vi "Repack Color to Color Array.vi"(11 "Pixel Data":T1={"A"=[0, 0, 0, 0, 0, 0, 0, 0], "R/H"=[0, 0, 0, 0, 0, 0, 0, 0], "G/S"=[0, 0, 0, 0, 0, 0, 0, 0], "B/L"=[0, 0, 0, 0, 0, 0, 0, 0]}) -> (3 "Output array U32x8":u32[](array[numeric]))   [LabVIEW 2017, in "NI_VDM_FPGA_Basics.lvlib"]
uses:
  <vilib>/visionFPGA/NI_VDM_FPGA_Basics.lvlib
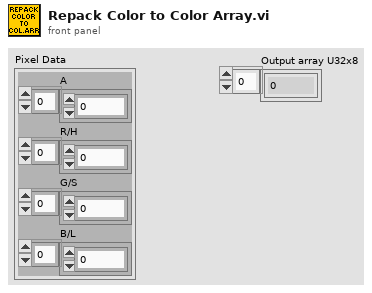
[diagram p1: front panel]
types:
  T1 = cluster{"A":u8[], "R/H":u8[], "G/S":u8[], "B/L":u8[]}
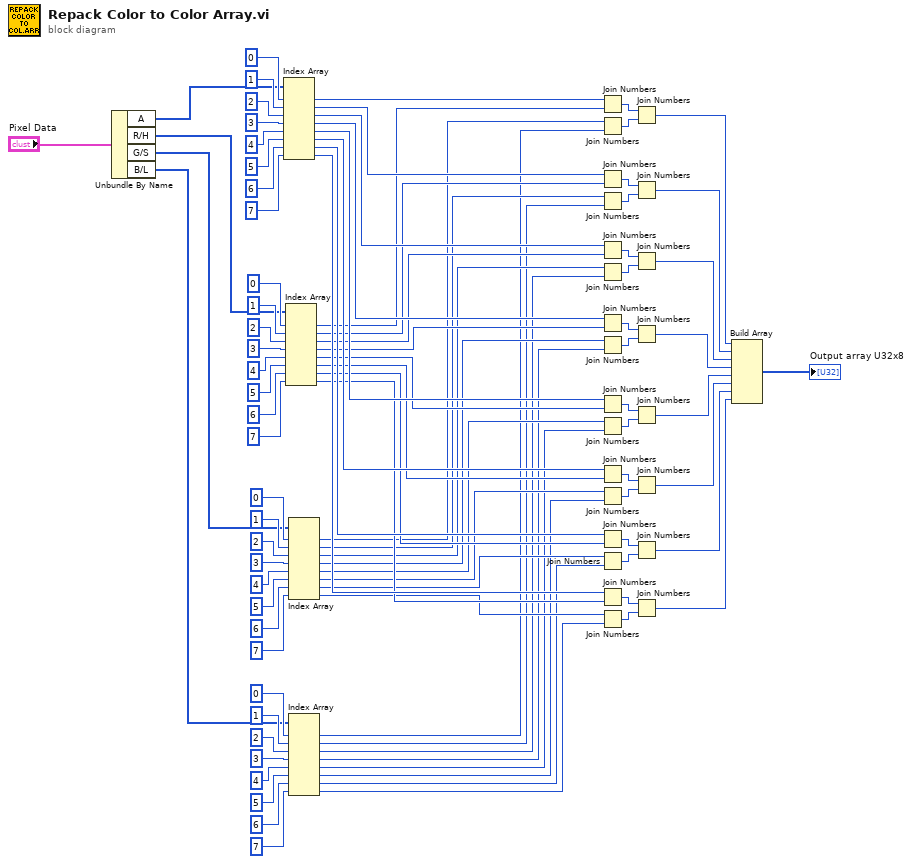
[diagram p0: block diagram]
diagram:
  n1 = Unbundle By Name("Pixel Data") -> ("A"=w85:u8[], "R/H"=w58:u8[], "G/S"=w57:u8[], "B/L"=w56:u8[])
  n2 = Index Array(array=w85, index #1=0 ("index"), index #2=1 ("index"), index #3=2 ("index"), index #4=3 ("index"), index #5=4 ("index"), index #6=5 ("index"), index #7=6 ("index"), index #8=7 ("index")) -> (element #1=w55:u8, element #2=w40:u8, element #3=w39:u8, element #4=w34:u8, element #5=w35:u8, element #6=w36:u8, element #7=w37:u8, element #8=w38:u8)
  n3 = Index Array(array=w58, index #1=0 ("index"), index #2=1 ("index"), index #3=2 ("index"), index #4=3 ("index"), index #5=4 ("index"), index #6=5 ("index"), index #7=6 ("index"), index #8=7 ("index")) -> (element #1=w33:u8, element #2=w32:u8, element #3=w31:u8, element #4=w30:u8, element #5=w29:u8, element #6=w28:u8, element #7=w27:u8, element #8=w26:u8)
  n4 = Index Array(array=w57, index #1=0 ("index"), index #2=1 ("index"), index #3=2 ("index"), index #4=3 ("index"), index #5=4 ("index"), index #6=5 ("index"), index #7=6 ("index"), index #8=7 ("index")) -> (element #1=w25:u8, element #2=w24:u8, element #3=w23:u8, element #4=w22:u8, element #5=w21:u8, element #6=w20:u8, element #7=w19:u8, element #8=w18:u8)
  n5 = Index Array(array=w56, index #1=0 ("index"), index #2=1 ("index"), index #3=2 ("index"), index #4=3 ("index"), index #5=4 ("index"), index #6=5 ("index"), index #7=6 ("index"), index #8=7 ("index")) -> (element #1=w17:u8, element #2=w16:u8, element #3=w15:u8, element #4=w14:u8, element #5=w13:u8, element #6=w12:u8, element #7=w11:u8, element #8=w10:u8)
  n6 = Join Numbers(hi=w55, lo=w33) -> ((hi.lo)=w84:u16)
  n7 = Join Numbers(hi=w25, lo=w17) -> ((hi.lo)=w83:u16)
  n8 = Join Numbers(hi=w40, lo=w32) -> ((hi.lo)=w53:u16)
  n9 = Join Numbers(hi=w24, lo=w16) -> ((hi.lo)=w54:u16)
  n10 = Join Numbers(hi=w39, lo=w31) -> ((hi.lo)=w52:u16)
  n11 = Join Numbers(hi=w23, lo=w15) -> ((hi.lo)=w51:u16)
  n12 = Join Numbers(hi=w34, lo=w30) -> ((hi.lo)=w49:u16)
  n13 = Join Numbers(hi=w22, lo=w14) -> ((hi.lo)=w50:u16)
  n14 = Join Numbers(hi=w35, lo=w29) -> ((hi.lo)=w48:u16)
  n15 = Join Numbers(hi=w21, lo=w13) -> ((hi.lo)=w47:u16)
  n16 = Join Numbers(hi=w36, lo=w28) -> ((hi.lo)=w45:u16)
  n17 = Join Numbers(hi=w20, lo=w12) -> ((hi.lo)=w46:u16)
  n18 = Join Numbers(hi=w37, lo=w27) -> ((hi.lo)=w44:u16)
  n19 = Join Numbers(hi=w19, lo=w11) -> ((hi.lo)=w43:u16)
  n20 = Join Numbers(hi=w38, lo=w26) -> ((hi.lo)=w41:u16)
  n21 = Join Numbers(hi=w18, lo=w10) -> ((hi.lo)=w42:u16)
  n22 = Join Numbers(hi=w84, lo=w83) -> ((hi.lo)=w9:u32)
  n23 = Join Numbers(hi=w53, lo=w54) -> ((hi.lo)=w8:u32)
  n24 = Join Numbers(hi=w52, lo=w51) -> ((hi.lo)=w7:u32)
  n25 = Join Numbers(hi=w49, lo=w50) -> ((hi.lo)=w6:u32)
  n26 = Join Numbers(hi=w48, lo=w47) -> ((hi.lo)=w5:u32)
  n27 = Join Numbers(hi=w45, lo=w46) -> ((hi.lo)=w4:u32)
  n28 = Join Numbers(hi=w44, lo=w43) -> ((hi.lo)=w3:u32)
  n29 = Join Numbers(hi=w41, lo=w42) -> ((hi.lo)=w2:u32)
  n30 = Build Array(w9, w8, w7, w6, w5, w4, w3, w2) -> (→"Output array U32x8":u32[])
